vi "ep_Read Single Line Wiring.vi"(8 "error in (no error)":errorcluster, 11 "system info in":refnum<class "EP System Info.lvclass">) -> (0 "error out":errorcluster, 2 "single line wiring? (F)":bool, 3 "system info out":refnum<class "EP System Info.lvclass">)   [LabVIEW 2014, in "NI_EP_Power Quality.lvlib" / "EP System Info.lvclass"]
uses:
  <vilib>/addons/Electrical Power/PQ/Common/Classes/System Info/EP System Info.lvclass
  <vilib>/addons/Electrical Power/PQ/Common/Classes/System Info/EP System Info.lvclass/EP System Info.ctl
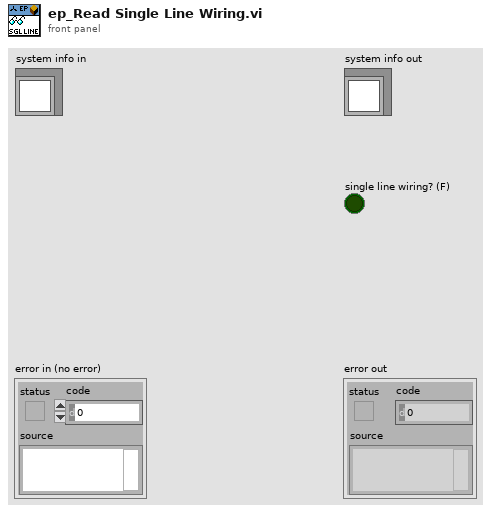
[diagram p1: front panel]
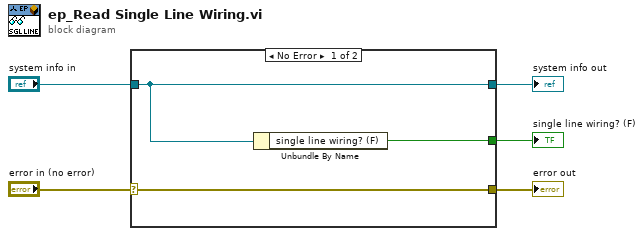
[diagram p0: block diagram]
diagram:
  n1 = case shown="No Error" "error in (no error)" {
    selector: "error in (no error)" -> [w8 w9]
    tunnel: [w8 w9] -> w4
    tunnel: [w7 w10] -> w2
    tunnel: "system info in" -> [w7 w10]
    tunnel: [w6 _] -> w1
    frame No Error {
      n2 = Unbundle By Name(w7) -> ("single line wiring? (F)"=w6:bool)
    }
    frame Error {
    }
  }
  "error out" <- w4
  "system info out" <- w2
  "single line wiring? (F)" <- w1
